vi "setStateValue.vi"(8 "error in (no error)":errorcluster, 10 "stateValue":string, 11 "ScriptEvent in":refnum<class "ScriptEvent.lvclass">) -> (0 "error out":errorcluster, 3 "ScriptEvent out":refnum<class "ScriptEvent.lvclass">)   [LabVIEW 2011, in "Tools.lvlib" / "Scripting.lvlib" / "ScriptEvent.lvclass"]
uses:
  ScriptEvent.lvclass
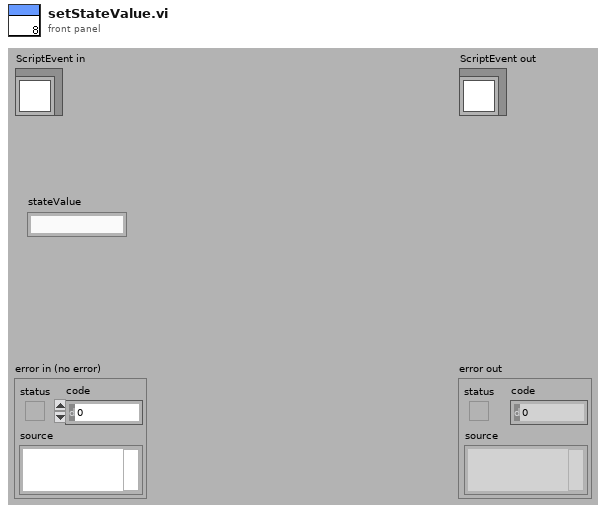
[diagram p1: front panel]
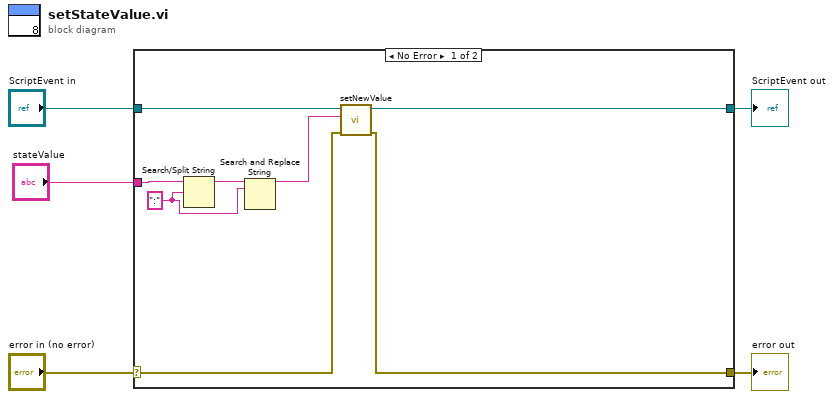
[diagram p0: block diagram]
diagram:
  n1 = case shown="No Error" "error in (no error)" {
    selector: "error in (no error)" -> [w8 w15]
    tunnel: [w7 w15] -> w4
    tunnel: [w9 w14] -> w2
    tunnel: "ScriptEvent in" -> [w12 w14]
    tunnel: "stateValue" -> [w13 _]
    frame No Error {
      w11 = ":"
      n2 = Search/Split String(string=w13, search string/char (-)=w11) -> (substring before match=w6:string)  [unwired: 1 in, 2 out]
      n3 = Search and Replace String(input string=w6, search string=w11) -> (result string=w10:string)  [unwired: 6 in, 3 out]
      n4 = call "setNewValue.vi"("error in (no error)"=w8, "newValue"=w10, "ScriptEvent.lvclass in"=w12) -> ("error out"=w7:errorcluster, "ScriptEvent.lvclass out"=w9:refnum<class "ScriptEvent.lvclass">)  [unwired: 7 in]
    }
    frame Error {
    }
  }
  "error out" <- w4
  "ScriptEvent out" <- w2
